vi "Read Config.vi"(8 "error in (no error)":errorcluster, 9 "Re-Init?":bool, 10 "ICM File In":path, 11 "NI Digital in":refnum<class "NI Analog Out.lvclass">) -> (0 "error out":errorcluster, 3 "NI Digital out":refnum<class "NI Analog Out.lvclass">)   [LabVIEW 2018, in "NI Analog Out.lvclass"]
doc: "NI Analog.lvclass:Read Config.vi\n\nThis VI reads the NI Analog Class parameters from the ICM configuration file.\n\nInstrument Communication Module Version 1.0\nJanuary, 2018 Original Code Consulting David Thomson\n www.originalcode.com"
uses:
  NI Analog Out.lvclass
  NI Analog Out.lvclass/NI Analog Out.ctl
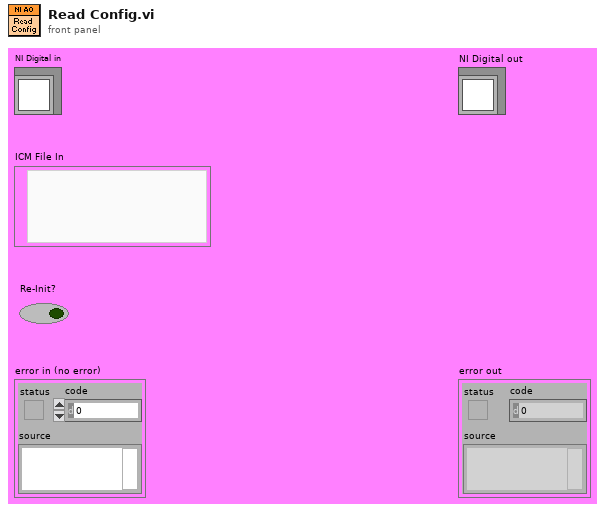
[diagram p1: front panel]
types:
  T1 = typedef "NI DO Type Def.ctl" = cluster{"Device":string, "SE/Diff":bool, "Channels":cluster{"Channel":i32, "Range":T2}[], "AD Write Time-out (s)":dbl}
  T2 = typedef "NI Analog Channel Range.ctl" = enum16{"-10.0 to 10.0 V", "-5.0 to 5.0 V", "-2.0 to 2.0 V", "-1.0 to 1.0 V", "-0.5 to 0.5 V", "-0.2 to 0.2 V", "-0.1 to 0.1 V", "0 to 10 V", "0 to 5 V", "0 to 2 V", "0 to 1 V", "0 to 0.5 V", "0 to 0.2 V", "0 to 0.1 V"}
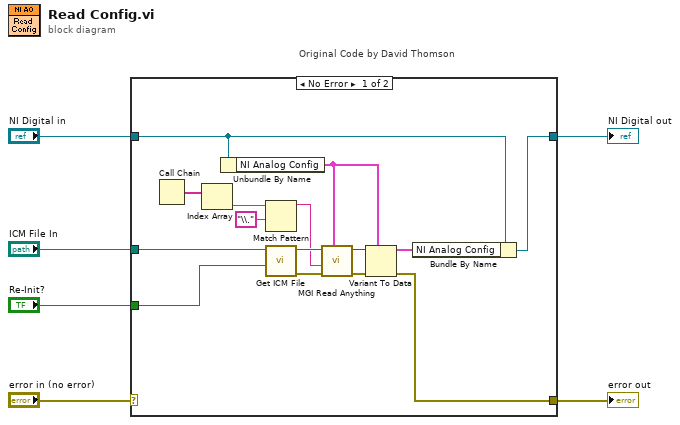
[diagram p0: block diagram]
diagram:
  n1 = case "Original Code by David Thomson" shown="No Error" "error in (no error)" {
    selector: "error in (no error)" -> [_ w23]
    tunnel: [w13 w23] -> w5
    tunnel: [w9 w22] -> w3
    tunnel: "NI Digital in" -> [w11 w22]
    tunnel: "ICM File In" -> [w8 _]
    tunnel: "Re-Init?" -> [w7 _]
    frame No Error {
      n2 = Call Chain() -> (call chain=w18:string[])
      n3 = Index Array(array=w18) -> (element=w19:string)  [unwired: 1 in]
      n4 = Unbundle By Name(w11) -> ("NI Analog Config"=w10:T1)
      n5 = Match Pattern(string=w19, regular expression="\\.") -> (before substring=w16:string)  [unwired: 1 in, 3 out]
      n6 = call "Get ICM File.vi"("Re-Init?"=w7, "ICM File In"=w8) -> ("error out"=w20:errorcluster, "ICM File"=w21:path)  [unwired: 8 in]
      n7 = call <userlib>:"MGI Read Anything.vi"("Type of Anything"=w10, "Error In"=w20, "Section Name (Name of \"Type of Anything\")"=w16, "Path (dialog)"=w21) -> ("Error Out"=w14:errorcluster, "Anything"=w15:variant)  [unwired: 4 in, 2 out]
      n8 = Variant To Data(error in=w14, type=w10, Variant=w15) -> (data=w12:T1, error out=w13:errorcluster)
      n9 = Bundle By Name(cluster=w11, "NI Analog Config"=w12) -> (w9:refnum<class "NI Analog Out.lvclass">)
    }
    frame Error {
    }
  }
  "error out" <- w5
  "NI Digital out" <- w3
